vi "VA_GenerateXYZ_withInputs.vi"(1 "Bias":dbl[](array[numeric]), 2 "Frequency":dbl=10.0, 3 "Amplitude":dbl[](array[numeric]), 4 "SampleFrequency":dbl=1000.0) -> (0 "xyz":dbl[](array[numeric]))   [LabVIEW 2011]
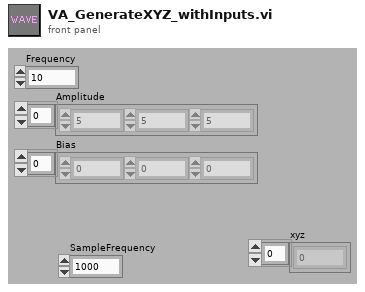
[diagram p1: front panel]
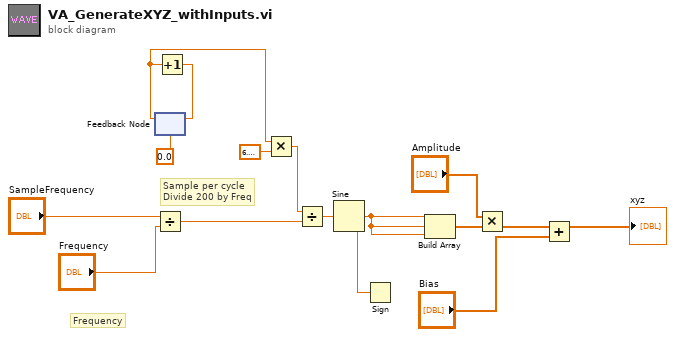
[diagram p0: block diagram]
diagram:
  # "Frequency"
  # "Sample per cycle\nDivide 200 by Freq"
  n1 = feedback #1(0.0) -> (w7:dbl)
  n2 = Divide(x="SampleFrequency", y="Frequency") -> (x/y=w11:dbl)
  n3 = Increment(x=w7) -> (x+1=w8:dbl)
  n4 = feedback-in #1(w8) -> ()
  n5 = Multiply(x=w7, y=6.283185307179586) -> (x*y=w14:dbl)
  n6 = Divide(x=w14, y=w11) -> (x/y=w13:dbl)
  n7 = Sine(x=w13) -> (sin(x)=w1:dbl)
  n8 = Sign(1:w1) -> ()  [unwired: 1 out]
  n9 = Build Array(w1, w1, w1) -> (w12:dbl[])
  n10 = Multiply(x="Amplitude", y=w12) -> (x*y=w5:dbl[])
  n11 = Add(x=w5, y="Bias") -> (x+y=→"xyz":dbl[])
